vi "ProdaNG.File.Export.PP.vi"(5 "Identification":T1, 6 "reason":string, 7 "TestStepsTree":refnum<vi>, 8 "error in (no error)":errorcluster, 10 "FileContent":T2, 11 "dbHandleIn":i32) -> (0 "error out":errorcluster, 3 "dbHandle":i32)   [LabVIEW 2016]
uses:
  ProdaNG.File.Sequence.ctl
  ProdaNG.Tree.Fglb.Value.ctl
  ProdaNG.File.Step.ctl
  ProdaNG.Tree.Fglb.Action.ctl
  ProdaNG.Tree.Fglb.Data.ctl
  ProdaNG.Tree.Fglb.Element.ctl
  ProdaNG.Configurator.Glb.vi
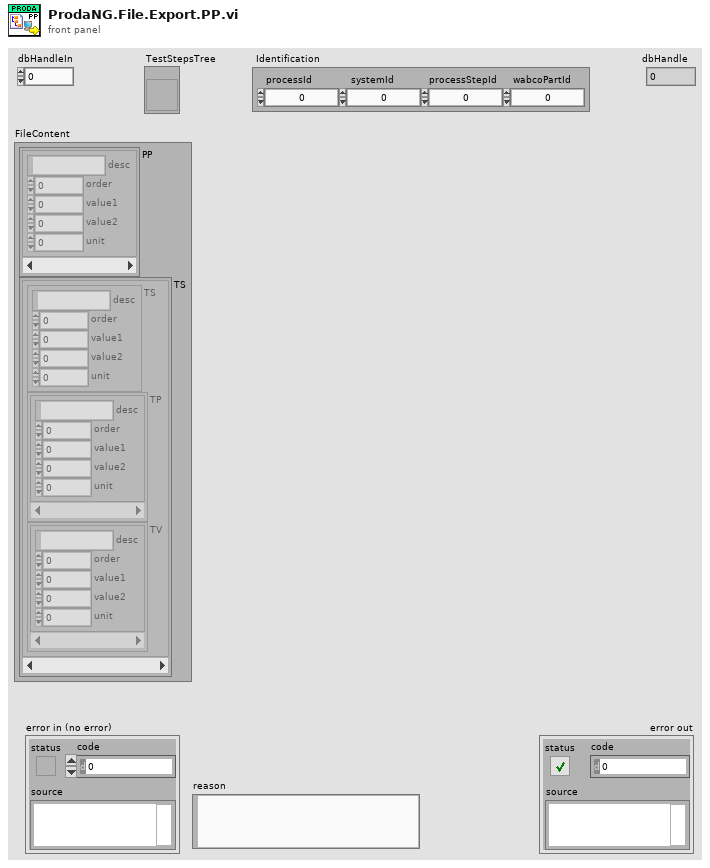
[diagram p1: front panel]
types:
  T1 = cluster{"processId":i32, "systemId":i32, "processStepId":i32, "wabcoPartId":i32}
  T2 = typedef "ProdaNG.File.Sequence.ctl" = cluster{"PP":T3[], "TS":T4[]}
  T3 = typedef "ProdaNG.Tree.Fglb.Value.ctl" = cluster{"desc":string, "order":i32, "value1":dbl, "value2":dbl, "unit":i32}
  T4 = typedef "ProdaNG.File.Step.ctl" = cluster{"TS":T3, "TP":T3[], "TV":T3[]}
  T5 = typedef "ProdaNG.Tree.Fglb.Data.ctl" = cluster{"tag":string, "row":i32, "element":T6, "idx1":i32, "idx2":i32, "file":bool}
  T6 = typedef "ProdaNG.Tree.Fglb.Element.ctl" = enum16{"-", "PP", "TS", "TP", "TV"}
  T7 = typedef "ProdaNG.Tree.Fglb.Action.ctl" = enum16{"init", "add", "get by row", "get by tag", "get by idx"}
  T8 = typedef "ProdaNG.ProcessStepParam.ctl" = cluster{"i_id":i32, "processStepId":i32, "unitId":i32, "contentId":string, "previewId":string, "value":dbl, "valueText":string, "paramSequence":i32, "history":i32, "mdReason":string, "mdUser":string, "mdTime":string, "description":string}
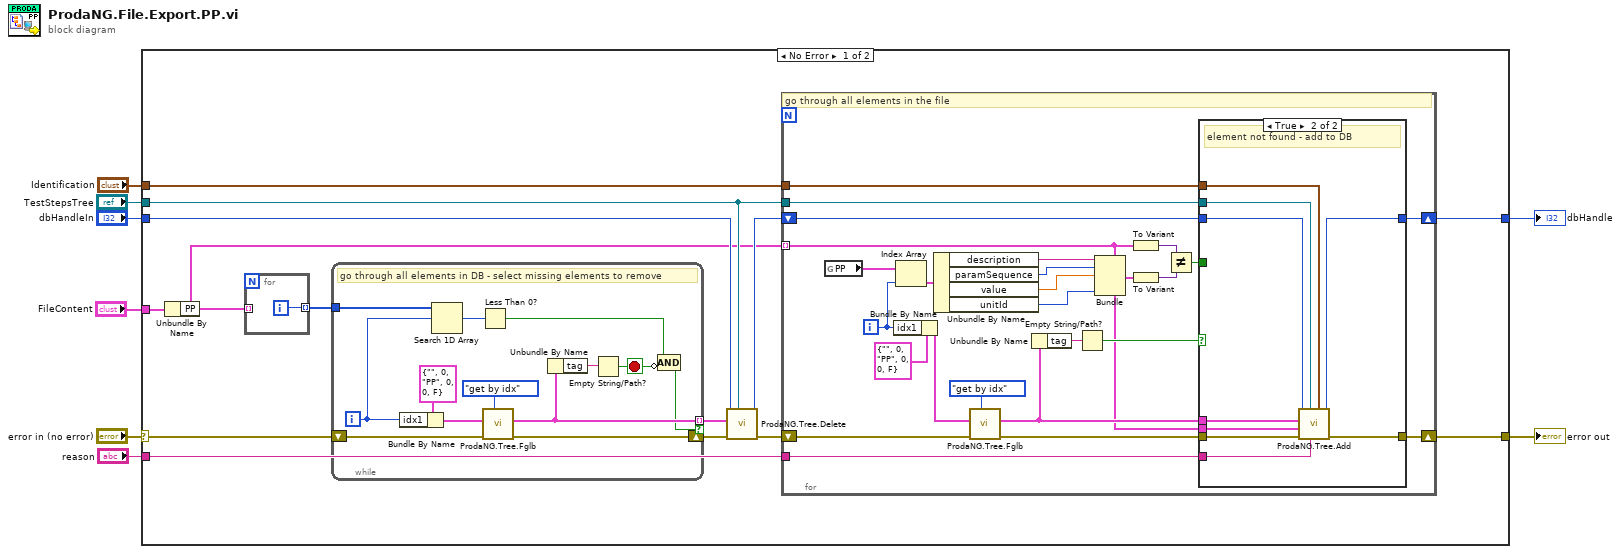
[diagram p0: block diagram]
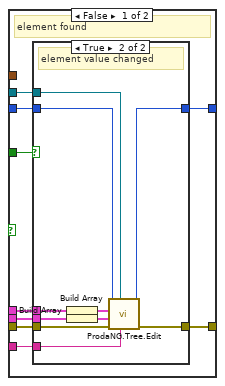
[diagram p2: hidden frame]
diagram:
  n1 = case shown="No Error" "error in (no error)" {
    selector: "error in (no error)" -> [w20 w94]
    tunnel: [w12 w94] -> w8
    tunnel: "dbHandleIn" -> [w15 w93]
    tunnel: [w22 w93] -> w5
    tunnel: "FileContent" -> [w21 _]
    tunnel: "reason" -> [w13 _]
    tunnel: "Identification" -> [w11 _]
    tunnel: "TestStepsTree" -> [w10 _]
    frame No Error {
      n2 = Unbundle By Name(w21) -> ("PP"=w9:T3[])
      n3 = for {
        tunnel: w9 -> [_] mode=indexing
        tunnel: [w23] -> w19 mode=indexing
        i -> [w23]
      }
      n4 = while {
        tunnel: [w32] -> w16 mode=indexing if=w28
        shift-right: [w31] -> w18
        shift-left: w20 -> [w35]
        tunnel: w19 -> [w30]
        i -> [w25]
        stop <- w24 stop-if-true
        # "go through all elements in DB - select missing elements to remove"
        n5 = Bundle By Name(cluster=T5 {"tag"="", "row"=0, "element"=enum."PP", "idx1"=0, "idx2"=0, "file"=FALSE} ("entry in"), "idx1"=w25) -> (w26:T5)
        n6 = Search 1D Array(1D array=w30, element=w25) -> (index of element=w29:i32)  [unwired: 1 in]
        n7 = Less Than 0?(x=w29) -> (x < 0?=w27:bool)
        n8 = call "ProdaNG.Tree.Fglb.vi"("Action (add)"=ProdaNG.Tree.Fglb.Action."get by idx", "error in"=w35, "entry in"=w26) -> ("error out"=w31:errorcluster, "found entry"=w32:T5)  [unwired: 6 in, 1 out]
        n9 = Unbundle By Name(w32) -> ("tag"=w33:string)
        n10 = Empty String/Path?(string/path=w33) -> (empty?=w24:bool)
        n11 = Compound Arithmetic op=AND(w27, invert w24) -> (w28:bool)
      }
      n12 = call "ProdaNG.Tree.Delete.vi"("TestStepsTree"=w10, "error in (no error)"=w18, "Elements to delete"=w16, "dbHandleIn"=w15) -> ("error out"=w17:errorcluster, "dbHandle"=w14:i32)  [unwired: 6 in]
      n13 = for {
        shift-right: [w54] -> w12
        shift-left: w17 -> [w59]
        shift-right: [w51] -> w22
        shift-left: w14 -> [w55]
        tunnel: w9 -> [w37] mode=indexing
        tunnel: w13 -> [w52]
        tunnel: w11 -> [w48]
        tunnel: w10 -> [w47]
        i -> [w38]
        # "go through all elements in the file"
        n14 = global read "ProdaNG.Configurator.Glb.vi" "PP"() -> (w50:T8[])
        n15 = Bundle By Name(cluster=T5 {"tag"="", "row"=0, "element"=enum."PP", "idx1"=0, "idx2"=0, "file"=FALSE} ("entry in"), "idx1"=w38) -> (w60:T5)
        n16 = Index Array(array=w50, index=w38) -> (element=w49:T8)
        n17 = Unbundle By Name(w49) -> ("description"=w46:string, "paramSequence"=w45:i32, "value"=w44:dbl, "unitId"=w43:i32)
        n18 = call "ProdaNG.Tree.Fglb.vi"("Action (add)"=ProdaNG.Tree.Fglb.Action."get by idx", "error in"=w59, "entry in"=w60) -> ("error out"=w56:errorcluster, "found entry"=w53:T5)  [unwired: 6 in, 1 out]
        n19 = Unbundle By Name(w53) -> ("tag"=w58:string)
        n20 = Empty String/Path?(string/path=w58) -> (empty?=w57:bool)
        n21 = Bundle(cluster=w37, "desc"=w46, "order"=w45, "value1"=w44, "unit"=w43) -> (w42:T3)  [unwired: 1 in]
        n22 = To Variant(anything=w37) -> (Variant=w41:variant)
        n23 = To Variant(anything=w42) -> (Variant=w40:variant)
        n24 = Not Equal?(x=w41, y=w40) -> (x != y?=w39:bool)
        n25 = case shown="True" w57 {
          tunnel: w56 -> [w71 w92]
          tunnel: w55 -> [w67 w91]
          tunnel: [w70 w86] -> w54
          tunnel: w53 -> [w68 w90]
          tunnel: w37 -> [w65 w89]
          tunnel: w52 -> [w69 w88]
          tunnel: [w66 w87] -> w51
          tunnel: w48 -> [_ w85]
          tunnel: w47 -> [w64 w84]
          tunnel: w39 -> [w63 _]
          frame False {
            # "element found"
            n26 = case shown="True" w63 {
              tunnel: w71 -> [w73 w83]
              tunnel: [w73 w82] -> w70
              tunnel: w69 -> [_ w81]
              tunnel: w68 -> [_ w80]
              tunnel: w67 -> [w72 w78]
              tunnel: [w72 w77] -> w66
              tunnel: w65 -> [_ w76]
              tunnel: w64 -> [_ w74]
              frame False {
              }
              frame True {
                # "element value changed"
                n27 = Build Array(w80) -> (w79:T5[])
                n28 = Build Array(w76) -> (w75:T3[])
                n29 = call "ProdaNG.Tree.Edit.vi"("reason"=w81, "TestStepsTree"=w74, "error in (no error)"=w83, "Selected elements values"=w75, "Selected elements"=w79, "dbHandleIn"=w78) -> ("error out"=w82:errorcluster, "dbHandle"=w77:i32)  [unwired: 4 in]
              }
            }
          }
          frame True {
            # "element not found - add to DB"
            n30 = call "ProdaNG.Tree.Add.vi"("Identification"=w85, "reason"=w88, "TestStepsTree"=w84, "error in (no error)"=w92, "Element values"=w89, "Element to add"=w90, "dbHandleIn"=w91) -> ("error out"=w86:errorcluster, "dbHandle"=w87:i32)  [unwired: 3 in]
          }
        }
      }
    }
    frame Error {
    }
  }
  "error out" <- w8
  "dbHandle" <- w5
